vi "TargetsDifferentCompilersMain.vi"   [LabVIEW 2019, in "TargetsDifferentCompilersLib.lvlib"]
uses:
  TargetsDifferentCompilersLib.lvlib
  Tests.Assets/ExternalDep/ExternalDepClass/ExternalDepClass.lvclass
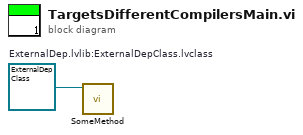
[diagram p0: block diagram]
diagram:
  w1 = refnum<class "ExternalDepClass.lvclass"> refnum  # ExternalDep.lvlib:ExternalDepClass.lvclass
  n1 = call-dynamic "SomeMethod.vi"("ExternalDepClass in"=w1) -> ()  [unwired: 9 in, 2 out]
